vi "Identity ID.vi"(11 "TaskTypeIdentity in":refnum<class "TaskTypeIdentity.lvclass">) -> (2 "ID":string)   [LabVIEW 2020, in "Volatus.lvlib" / "TaskTypeIdentity.lvclass"]
uses:
  TaskTypeIdentity.lvclass
  TaskTypeIdentity.lvclass/TaskTypeIdentity.ctl
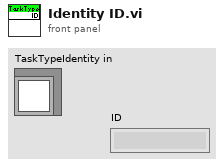
[diagram p1: front panel]
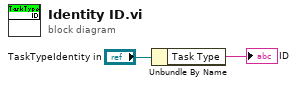
[diagram p0: block diagram]
diagram:
  n1 = Unbundle By Name("TaskTypeIdentity in") -> ("Task Type"=→"ID":string)
